vi "Get_ref_inst_value.vi"(0 "Ref Instrument type":T2, 2 "ADAM Channel Name":string, 7 "Index in":i32, 9 "Velocity Cluster Array":T1[](array[typedef])=[{"Name"="", "U"=0.0, "u^2"=0.0, "u^3/(u^2)^(1.5)"=0.0, "u^4/(u^2)^2 -3"=0.0, "% u'/U"=0.0, "Mean % Err"=0.0, "u^4"=0.0}, {"Name"="", "U"=0.0, "u^2"=0.0, "u^3/(u^2)^(1.5)"=0.0, "u^4/(u^2)^2 -3"=0.0, "% u'/U"=0.0, "Mean % Err"=0.0, "u^4"=0.0}, {"Name"="", "U"=0.0, "u^2"=0.0, "u^3/(u^2)^(1.5)"=0.0, "u^4/(u^2)^2 -3"=0.0, "% u'/U"=0.0, "Mean % Err"=0.0, "u^4"=0.0}, {"Name"="", "U"=0.0, "u^2"=0.0, "u^3/(u^2)^(1.5)"=0.0, "u^4/(u^2)^2 -3"=0.0, "% u'/U"=0.0, "Mean % Err"=0.0, "u^4"=0.0}] {"u^4" format="%.2f"; "Mean % Err" format="%.2f"; "u^4/(u^2)^2 -3" format="%.2f"; "u^3/(u^2)^(1.5)" format="%.2f"; "u^2" format="%.2f"; "% u'/U" format="%.2f"; "U" format="%.2f"}, 13 "Start time":dbl format="%.2f") -> (4 "Ref Value":dbl format="%.2f", 10 "Index out":i32)   [LabVIEW 2010]
uses:
  Controls/Ref_Inst_type.ctl
  Controls/Velocity_cluster.ctl
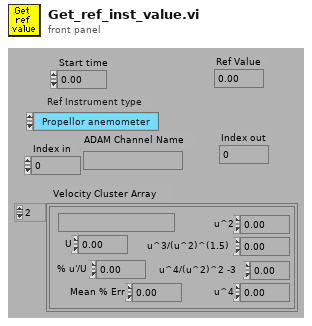
[diagram p1: front panel]
types:
  T1 = typedef "Velocity_cluster.ctl" = cluster{"Name":string, "U":dbl, "u^2":dbl, "u^3/(u^2)^(1.5)":dbl, "u^4/(u^2)^2 -3":dbl, "% u'/U":dbl, "Mean % Err":dbl, "u^4":dbl}
  T2 = typedef "Ref_Inst_type.ctl" = enum16{"Propellor anemometer", "Pressure Transducer", "Raw voltage", "Pitot-static tube", "Preston tube", "Generic Linear", "Generic Polynomial", "Thermocouple", "LDA", "Enter Value", "ADAM Channel"}
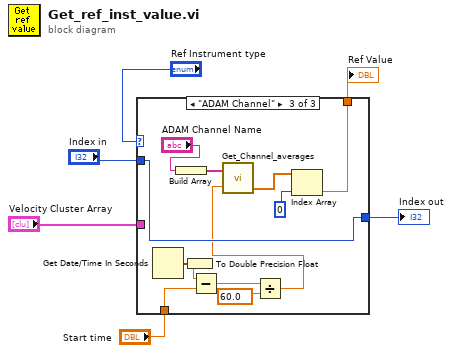
[diagram p0: block diagram]
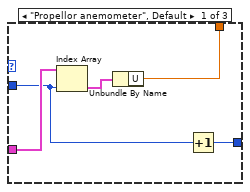
[diagram p2: hidden frame]
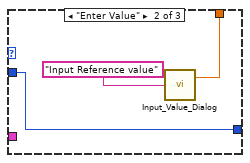
[diagram p3: hidden frame]
diagram:
  n1 = case shown="\"ADAM Channel\"" "Ref Instrument type" {
    tunnel: [w9 w14 w17] -> w4
    tunnel: "Index in" -> [w8 w12 w26]
    tunnel: "Start time" -> [_ _ w23]
    tunnel: "Velocity Cluster Array" -> [w11 _ _]
    tunnel: [w7 w12 w26] -> w2
    frame "Propellor anemometer", Default {
      n2 = Index Array(array=w11, index=w8) -> (element=w10:T1)
      n3 = Unbundle By Name(w10) -> ("U"=w9:dbl)
      n4 = Increment(x=w8) -> (x+1=w7:i32)
    }
    frame "Enter Value" {
      n5 = call "Input_Value_Dialog.vi"("Message to user"="Input Reference value") -> ("Value received"=w14:dbl)  [unwired: 1 out]
    }
    frame "ADAM Channel" {
      n6 = Get Date/Time In Seconds() -> (seconds since 1Jan1904=w16:timestamp)
      n7 = Build Array("ADAM Channel Name") -> (w25:string[])
      n8 = To Double Precision Float(number=w16) -> (double precision float=w24:dbl)
      n9 = Subtract(x=w24, y=w23) -> (x-y=w22:dbl)
      n10 = Divide(x=w22, y=60.0) -> (x/y=w20:dbl)
      n11 = call "Get_Channel_averages.vi"("Desired Ch Names"=w25, "Averaging time (mins)"=w20) -> ("number"=w19:dbl[])  [unwired: 1 in, 2 out]
      n12 = Index Array(array=w19, index=0 ("Index")) -> (element=w17:dbl)
    }
  }
  "Index out" <- w2
  "Ref Value" <- w4
